vi "Get SA Pin.vi"(8 "error in (no error)":errorcluster, 11 "NF in":refnum<class "NF.lvclass">) -> (0 "error out":errorcluster, 2 "SA Pin":string, 3 "NF out":refnum<class "NF.lvclass">)   [LabVIEW 2018, in "NF.lvlib" / "NF.lvclass"]
uses:
  NF.lvclass
  C:/Sequence Automation/Plugins/Measurement Interface.lvlibp/Measurement Interface.lvclass
  Plugins/Measurement Interface.lvlibp/Private Methods/Measurement Parameters/Read Measurement Parameters.vi
  Plugins/String Database.lvlibp/String Database.lvclass
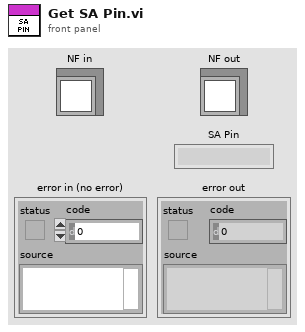
[diagram p1: front panel]
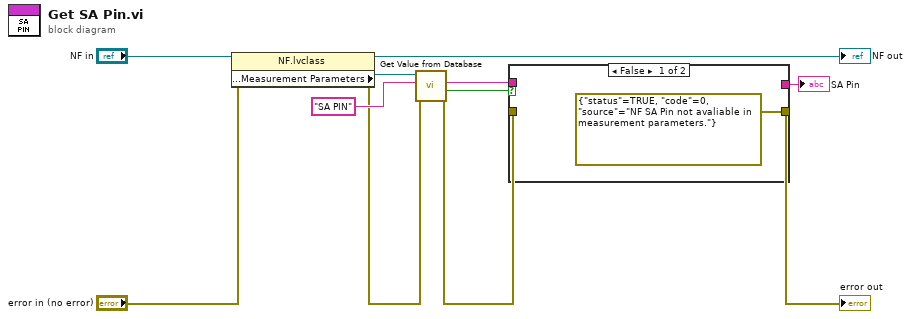
[diagram p0: block diagram]
diagram:
  n1 = property class="NF.lvclass"(reference="NF in", error in="error in (no error)") -> (reference out=→"NF out":refnum<class "NF.lvclass">, error out=w9:errorcluster, "Protected Methods:Measurement Parameters"=w11:refnum<class "String Database.lvclass">)
  n2 = call "Get Value from Database.vi"("error in (no error)"=w9, "Entry Name"="SA PIN", "Message in"=w11) -> ("error out"=w7:errorcluster, "Entry Found"=w8:bool, "Entry Value"=w6:string)  [unwired: 5 in, 1 out]
  n3 = case shown="False" w8 {
    tunnel: w7 -> [_ w13]
    tunnel: [errorcluster {"status"=TRUE, "code"=0, "source"="NF SA Pin not avaliable in measurement parameters."} ("error out") w13] -> w1
    tunnel: w6 -> [_ w14]
    tunnel: [_ w14] -> w5
    frame False {
    }
    frame True {
    }
  }
  "error out" <- w1
  "SA Pin" <- w5
